vi "纳清pH_所有参数读取.vi"(8 "error in (no error)":errorcluster caption="错误输入（无错误）", 11 "MB session in":refnum<class "MB_Master.lvclass">) -> (0 "error out":errorcluster caption="错误输出", 2 "输出值":T1 {"波特率" items=["4800", "9600", "19200", "38400", "57600", "115200"]}, 3 "MB session out":refnum<class "MB_Master.lvclass">)   [LabVIEW 2016, in "斯坦道多参数.lvlib"]
uses:
  <vilib>/Plasmionique/MB Master/MB_Master/MB_Master.lvclass
  <vilib>/Plasmionique/MB Master/MB Master.lvlib
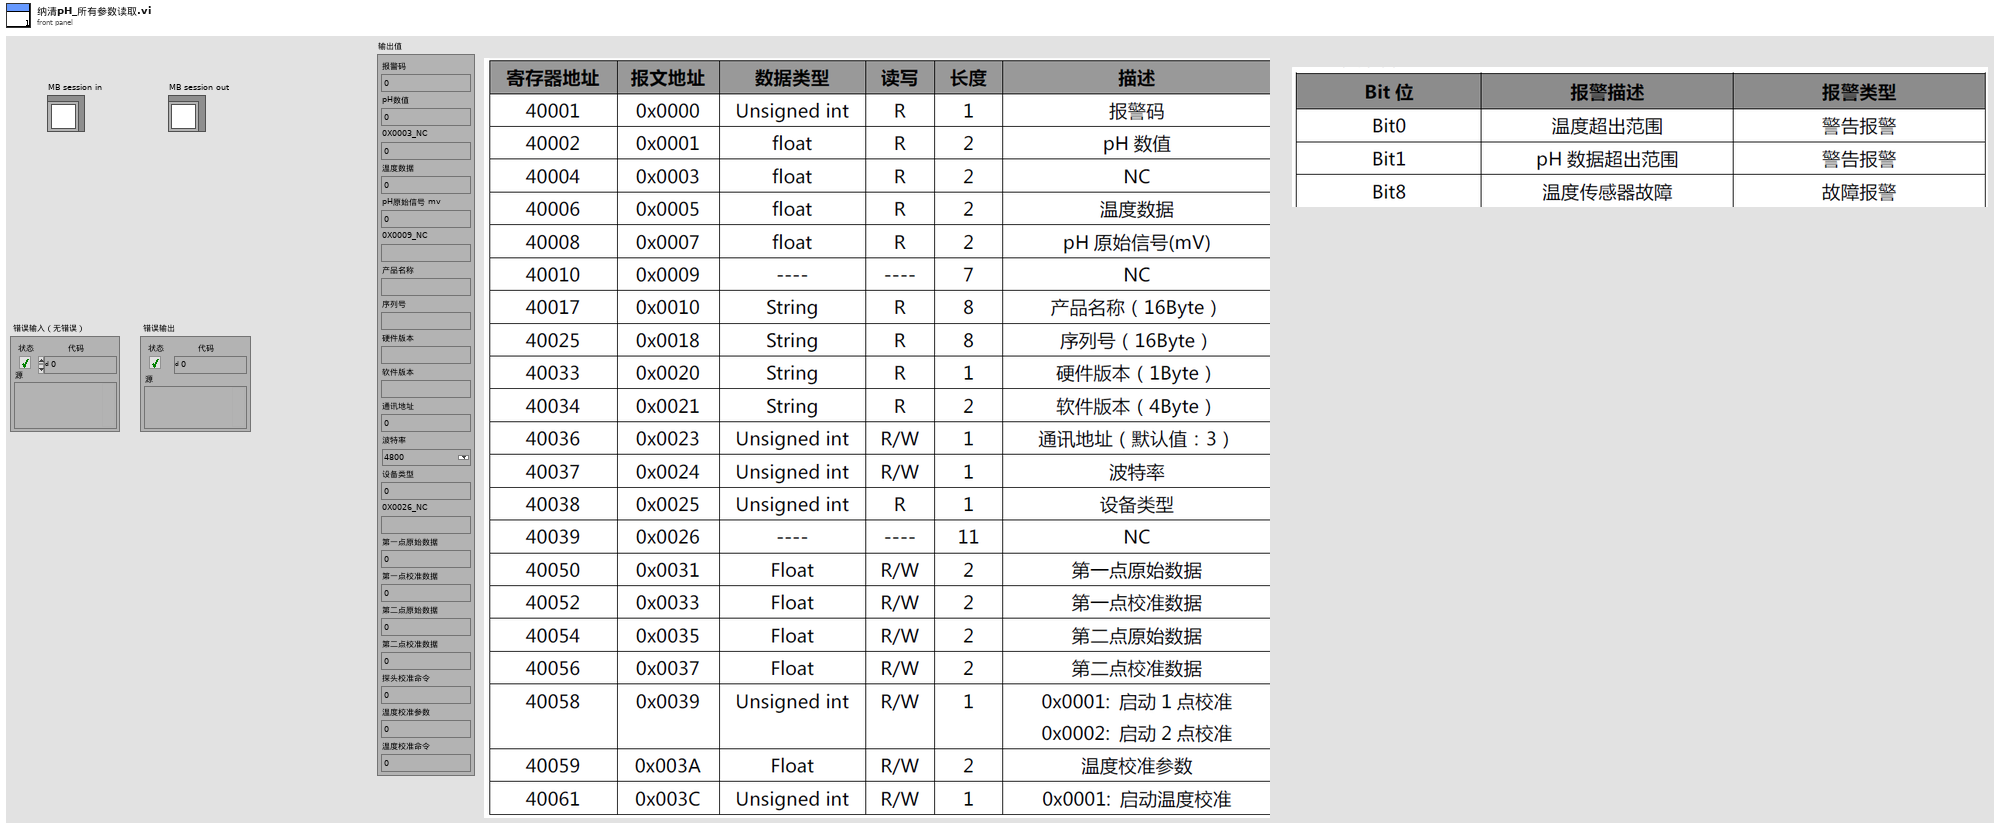
[diagram p1: front panel]
types:
  T1 = cluster{"报警码":u16, "pH数值":sgl, "0X0003_NC":sgl, "温度数据":sgl, "pH原始信号 mv":sgl, "0X0009_NC":string, "产品名称":string, "序列号":string, "硬件版本":string, "软件版本":string, "通讯地址":u16, "波特率":u16, "设备类型":u16, "0X0026_NC":string, "第一点原始数据":sgl, "第一点校准数据":sgl, "第二点原始数据":sgl, "第二点校准数据":sgl, "探头校准命令":u16, "温度校准参数":sgl, "温度校准命令":u16}
  T2 = cluster{u16, "数值":sgl, "数值":sgl, "数值":sgl, "数值":sgl, "类型":string, "类型":string, "类型":string, "类型":string, "类型":string, u16, u16, u16, "类型":string, "数值":sgl, "数值":sgl, "数值":sgl, "数值":sgl, u16, "数值":sgl, u16}
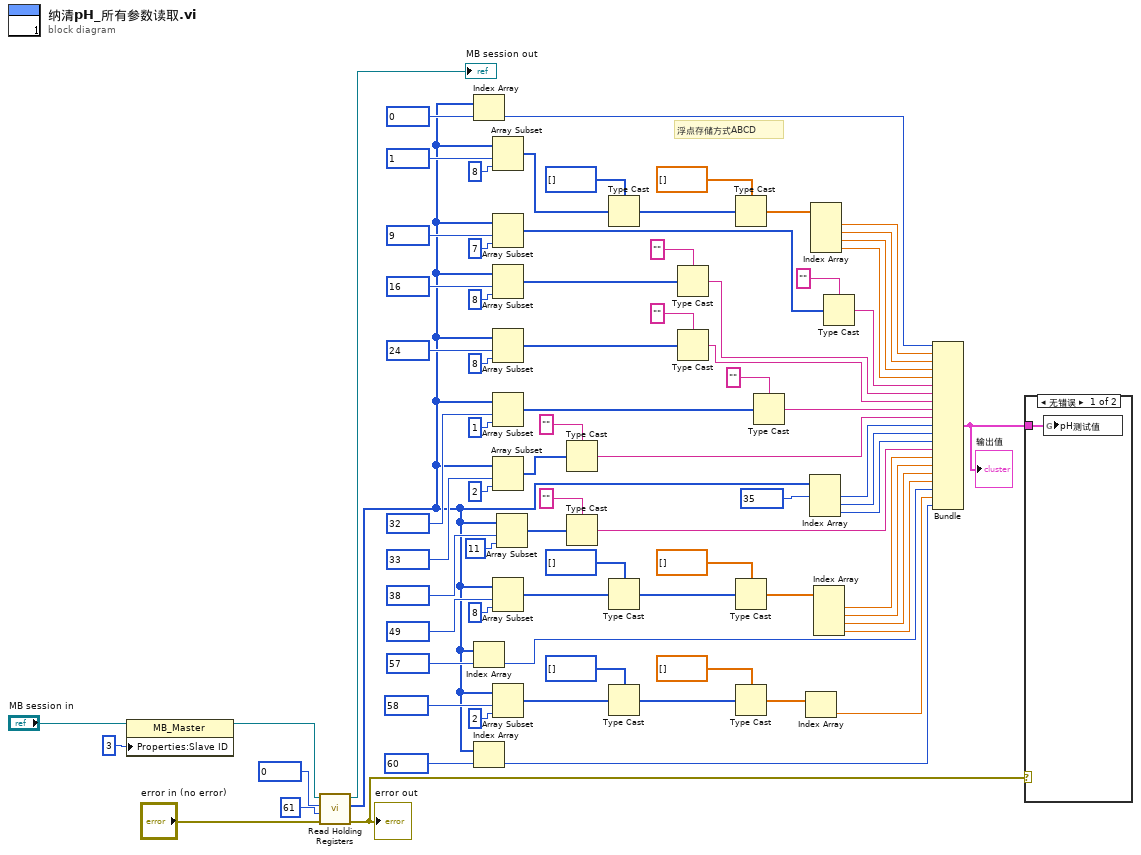
[diagram p0: block diagram]
diagram:
  # "浮点存储方式ABCD"
  n1 = property class="MB_Master"(reference="MB session in", "Properties:Slave ID"=u8 3 ("Slave ID")) -> (reference out=w70:refnum<class "MB_Master.lvclass">)  [unwired: 1 in, 1 out]
  n2 = call <vilib>:"Read Holding Registers.vi"("error in (no error)"="error in (no error)", "quantity"=u16 61, "starting address"=u16 0, "MB session in"=w70) -> ("error out"=w10:errorcluster, "Registers"=w12:u16[], "MB session out"=→"MB session out":refnum<class "MB_Master.lvclass">)  [unwired: 5 in]
  "error out" <- w10
  n3 = Index Array(array=w12, index=u16 0 ("starting address")) -> (element=w78:u16)
  n4 = Index Array(array=w12, index=u16 57 ("starting address")) -> (element=w15:u16)
  n5 = Index Array(array=w12, index=u16 60 ("starting address")) -> (element=w11:u16)
  n6 = Array Subset(array=w12, index=u16 1 ("starting address"), length=8 ("长度")) -> (w74:u16[])
  n7 = Array Subset(array=w12, index=u16 9 ("starting address"), length=7 ("长度")) -> (w63:u16[])
  n8 = Array Subset(array=w12, index=u16 16 ("starting address"), length=8 ("长度")) -> (w59:u16[])
  n9 = Array Subset(array=w12, index=u16 24 ("starting address"), length=8 ("长度")) -> (w53:u16[])
  n10 = Array Subset(array=w12, index=u16 32 ("starting address"), length=1 ("长度")) -> (w49:u16[])
  n11 = Array Subset(array=w12, index=u16 33 ("starting address"), length=2 ("长度")) -> (w43:u16[])
  n12 = Array Subset(array=w12, index=u16 49 ("starting address"), length=8 ("长度")) -> (w30:u16[])
  n13 = Array Subset(array=w12, index=u16 58 ("starting address"), length=2 ("长度")) -> (w18:u16[])
  n14 = Array Subset(array=w12, index=u16 38 ("starting address"), length=11 ("长度")) -> (w33:u16[])
  n15 = Type Cast(type="" ("类型"), x=w43) -> (*(type *) &x=w41:string)
  n16 = Type Cast(type="" ("类型"), x=w33) -> (*(type *) &x=w32:string)
  n17 = Type Cast(type=u32[] [] ("数组 2"), x=w74) -> (*(type *) &x=w9:u32[])
  n18 = Type Cast(type=u32[] [] ("数组 2"), x=w30) -> (*(type *) &x=w28:u32[])
  n19 = Type Cast(type=u32[] [] ("数组 2"), x=w18) -> (*(type *) &x=w20:u32[])
  n20 = Type Cast(type="" ("类型"), x=w59) -> (*(type *) &x=w56:string)
  n21 = Type Cast(type="" ("类型"), x=w53) -> (*(type *) &x=w51:string)
  n22 = Type Cast(type=sgl[] [] ("数组 2"), x=w9) -> (*(type *) &x=w73:sgl[])
  n23 = Type Cast(type=sgl[] [] ("数组 2"), x=w28) -> (*(type *) &x=w25:sgl[])
  n24 = Type Cast(type=sgl[] [] ("数组 2"), x=w20) -> (*(type *) &x=w23:sgl[])
  n25 = Type Cast(type="" ("类型"), x=w49) -> (*(type *) &x=w46:string)
  n26 = Index Array(array=w23) -> (element=w14:sgl)  [unwired: 1 in]
  n27 = Index Array(array=w12, index #1=u16 35 ("starting address")) -> (element #1=w39:u16, element #2=w38:u16, element #3=w37:u16)  [unwired: 2 in]
  n28 = Index Array(array=w73) -> (element #1=w68:sgl, element #2=w67:sgl, element #3=w6:sgl, element #4=w5:sgl)  [unwired: 4 in]
  n29 = Index Array(array=w25) -> (element #1=w24:sgl, element #2=w4:sgl, element #3=w3:sgl, element #4=w2:sgl)  [unwired: 4 in]
  n30 = Type Cast(type="" ("类型"), x=w63) -> (*(type *) &x=w61:string)
  n31 = Bundle(w78, "数值"=w68, "数值"=w67, "数值"=w6, "数值"=w5, "类型"=w61, "类型"=w56, "类型"=w51, "类型"=w46, "类型"=w41, w39, w38, w37, "类型"=w32, "数值"=w24, "数值"=w4, "数值"=w3, "数值"=w2, w15, "数值"=w14, w11) -> (w1:T2)  [unwired: 1 in]
  "输出值" <- w1
  n32 = case shown="无错误" w10 {
    tunnel: w1 -> [w81 _]
    frame No Error {
      n33 = global write "纳清过程全局变量.vi" "pH测试值"(w81) -> ()
    }
    frame Error {
    }
  }
